vi "Image name -- FGV.vi"(8 "error in (no error)":errorcluster, 10 "Action":T1, 11 "Base name":path=path "Image_") -> (0 "error out":errorcluster, 3 "Path out":path)   [LabVIEW 2020]
uses:
  controls/FGV actions -- enum.ctl
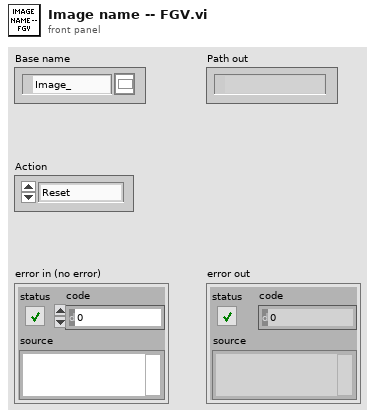
[diagram p1: front panel]
types:
  T1 = typedef "FGV actions -- enum.ctl" = enum16{"Reset", "Get", "Increment"}
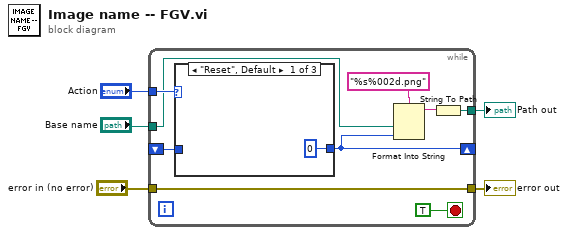
[diagram p0: block diagram]
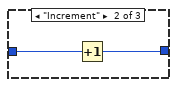
[diagram p2: hidden frame]
diagram:
  n1 = while {
    tunnel: "Action" -> [w13]
    shift-right: [w10] -> _
    shift-left: _ -> [w12]
    tunnel: "Base name" -> [w11]
    tunnel: [w7] -> w5
    tunnel: "error in (no error)" -> [w6]
    tunnel: [w6] -> w1
    stop <- TRUE stop-if-true
    n2 = case shown="\"Reset\", Default" w13 {
      tunnel: w12 -> [_ w17 w18]
      tunnel: [0 w16 w18] -> w10
      frame "Reset", Default {
      }
      frame "Increment" {
        n3 = Increment(x=w17) -> (x+1=w16:i32)
      }
      frame "Get" {
      }
    }
    n4 = Format Into String(format string="%s%002d.png", w11, w10) -> (resulting string=w8:string)  [unwired: 2 in, 1 out]
    n5 = String To Path(string=w8) -> (path=w7:path)
  }
  "Path out" <- w5
  "error out" <- w1
